vi "TestGetMeasures.vi"() -> ()   [LabVIEW 2019]
uses:
  ByteGSAPIBase.lvclass
panel:
  in  "Tree":string(tree)
  out "Meas":sgl[](graph)
  out "error out":errorcluster
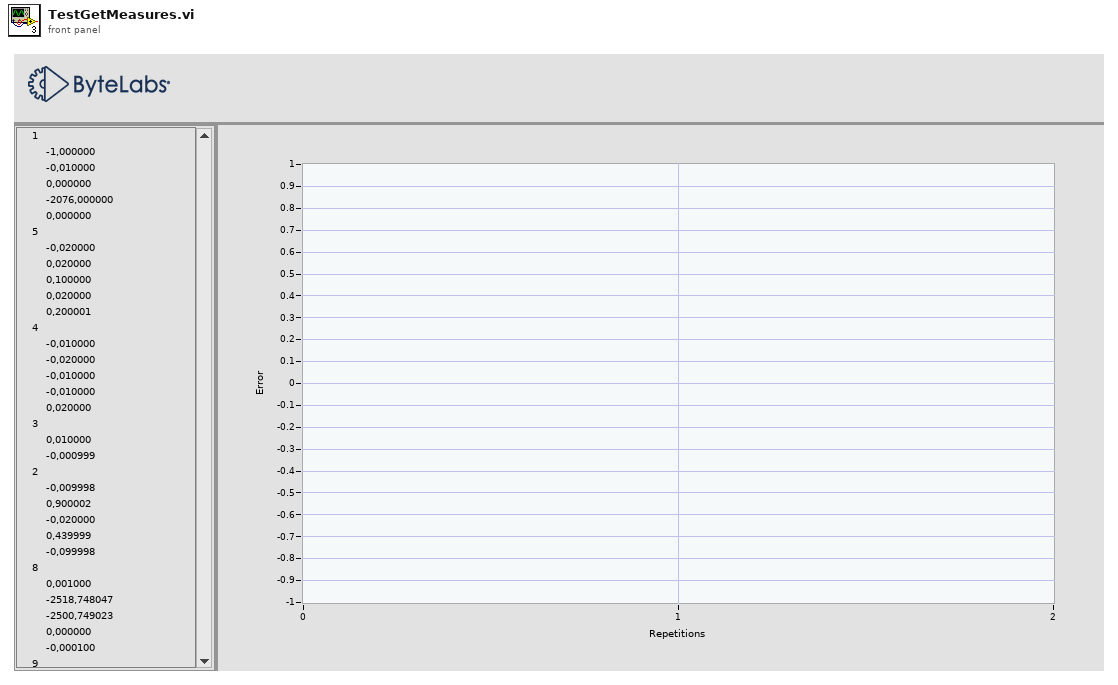
[diagram p1: front panel]
types:
  T1 = typedef "ByteGSWebAPI.lvlib/ByteGSAPIBase.lvclass/EditMeasurementReqData.ctl" = cluster{"misura_strumento":sgl}
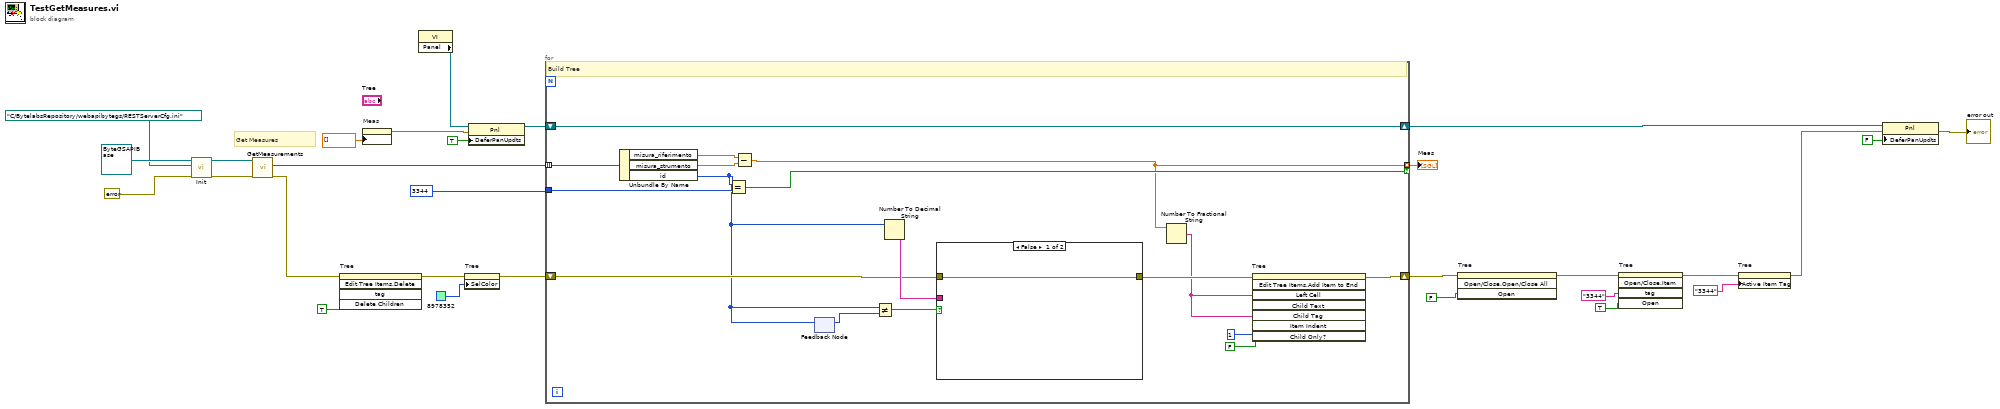
[diagram p0: block diagram]
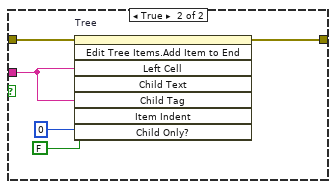
[diagram p2: hidden frame]
diagram:
  # "Get Measures"
  n1 = call-dynamic "Init.vi"("error in (no error)"=errorcluster {"status"=FALSE, "code"=0, "source"=""}, "Server cfg"=path "C:/BytelabsRepository/webapibytegs/RESTServerCfg.ini" ("configuration file path"), "ByteGSAPIBase in"=refnum<class "ByteGSAPIBase.lvclass"> refnum ("ByteGSWebAPI.lvlib:ByteGSAPIBase.lvclass")) -> ("error out"=w25:errorcluster, "ByteGSAPIBase out"=w26:refnum<class "ByteGSAPIBase.lvclass">)  [unwired: 7 in]
  n2 = call-dynamic "GetMeasurements.vi"("error in (no error)"=w25, "ByteGSAPIBase in"=w26) -> ("error out"=w19:errorcluster, "Array"=w24:T1[])  [unwired: 7 in, 1 out]
  n3 = invoke on="Tree" class="Tree (strict)" method="Edit Tree Items.Delete"(error in=w19, "Delete Children"=TRUE ("Delete Children?")) -> (error out=w11:errorcluster)  [unwired: 3 in, 4 out]
  n4 = property on="Meas" class="WFChart (strict)"("History Data"=sgl[] []) -> (error out=w17:errorcluster)  [unwired: 2 in, 1 out]
  n5 = property class="VI"() -> ("Panel"=w18:refnum<vi>)  [unwired: 2 in, 2 out]
  n6 = property on="Tree" class="Tree (strict)"(error in=w11, "SelColor"=u32 8978352) -> (error out=w10:errorcluster)  [unwired: 1 in, 1 out]
  n7 = property class="Pnl"(reference=w18, error in=w17, "DeferPanUpdts"=TRUE ("Defer Panel Updates")) -> (reference out=w15:refnum<vi>)  [unwired: 1 out]
  n8 = for {
    tunnel: w24 -> [w46] mode=indexing
    tunnel: u16 3344 ("IdMeas") -> [w45]
    tunnel: [w38] -> w22 mode=indexing if=w44
    shift-right: [w35] -> w7
    shift-left: w10 -> [w36]
    shift-right: [w30] -> w14
    shift-left: w15 -> [w30]
    # "Build Tree"
    n9 = Unbundle By Name(w46) -> ("misura_riferimento"=w43:sgl, "misura_strumento"=w42:sgl, "id"=w32:u16)
    n10 = Equal?(x=w32, y=w45) -> (x = y?=w44:bool)
    n11 = Subtract(x=w43, y=w42) -> (x-y=w38:sgl)
    n12 = feedback-in #1(w32) -> ()
    n13 = feedback #1() -> (w31:u16)  [unwired: 1 in]
    n14 = Not Equal?(x=w32, y=w31) -> (x != y?=w33:bool)
    n15 = Number To Decimal String(number=w32) -> (decimal integer string=w41:string)  [unwired: 1 in]
    n16 = case shown="False" w33 {
      tunnel: w41 -> [_ w51]
      tunnel: [w47 w50] -> w40
      tunnel: w36 -> [w47 w48]
      frame False {
      }
      frame True {
        n17 = invoke on="Tree" class="Tree (strict)" method="Edit Tree Items.Add Item to End"(error in=w48, "Left Cell"=w51, "Child Tag"=w51, "Item Indent"=0 ("New Item Indentation"), "Child Only?"=FALSE) -> (error out=w50:errorcluster)  [unwired: 3 in, 7 out]
      }
    }
    n18 = Number To Fractional String(number=w38) -> (F-format string=w34:string)  [unwired: 3 in]
    n19 = invoke on="Tree" class="Tree (strict)" method="Edit Tree Items.Add Item to End"(error in=w40, "Left Cell"=w34, "Child Tag"=w34, "Item Indent"=1 ("New Item Indentation"), "Child Only?"=FALSE) -> (error out=w35:errorcluster)  [unwired: 3 in, 7 out]
  }
  "Meas" <- w22
  n20 = invoke on="Tree" class="Tree (strict)" method="Open/Close.Open/Close All"(error in=w7, "Open"=FALSE ("Open?")) -> (error out=w6:errorcluster)  [unwired: 2 in, 3 out]
  n21 = invoke on="Tree" class="Tree (strict)" method="Open/Close.Item"(error in=w6, "tag"="3344" ("Tag"), "Open"=TRUE ("Open?")) -> (error out=w3:errorcluster)  [unwired: 2 in, 4 out]
  n22 = property on="Tree" class="Tree (strict)"(error in=w3, "Active Item Tag"="3344" ("Tag")) -> (error out=w1:errorcluster)  [unwired: 1 in, 1 out]
  n23 = property class="Pnl"(reference=w14, error in=w1, "DeferPanUpdts"=FALSE ("Defer Panel Updates")) -> (error out=→"error out":errorcluster)  [unwired: 1 out]
